vi "Load Settings from XML.vi"() -> (0 "error out":errorcluster, 3 "Settings Out":T1 {"Units" items=["degC", "degF", "kelvin", "raw"]})   [LabVIEW 2020, in "Settings Editor.lvlib"]
doc: "Attempts to load previous user specified settings from an XML file.\n\nThis VI will not generate an error. If a suitable XML file can't be loaded and parsed then it will simply return the default settings.\n_____\nBased on Delacor QMH Project Template 5.0.0.82."
uses:
  Settings Editor.lvlib
  Settings--cluster.ctl
  <vilib>/Utility/xml.llb/Read From XML File(string).vi
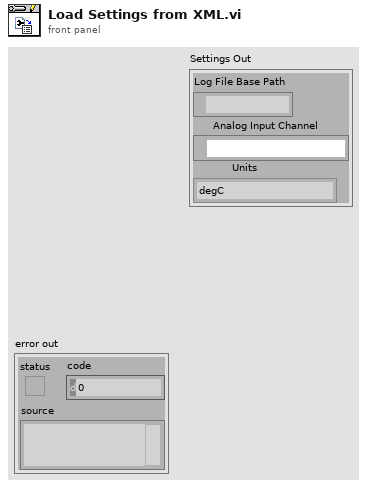
[diagram p1: front panel]
types:
  T1 = typedef "Settings Editor.lvlib/Settings--cluster.ctl" = cluster{"Log File Base Path":path, "Analog Input Channel":refnum<k21>, "Units":i32}
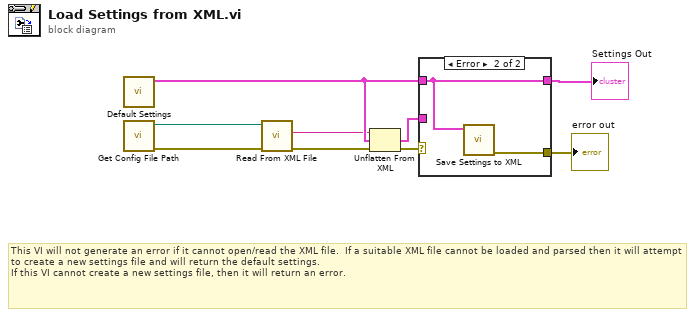
[diagram p0: block diagram]
diagram:
  # "This VI will not generate an error if it cannot open/read the XML file.  If a suitable XML file cannot be loaded and parsed then it will attempt to create a new settings file and will return the default settings.\nIf this VI cannot create a new settings file, then it will return an error."
  n1 = call "Default Settings.vi"() -> ("Default Settings"=w8:T1)  [unwired: 11 in]
  n2 = call "Get Config File Path.vi"() -> ("error out"=w4:errorcluster, "XML File Path"=w5:path)  [unwired: 10 in]
  n3 = call-poly <vilib>:"Read From XML File.vi"("error in (no error)"=w4, "XML File Path"=w5) -> ("error out"=w6:errorcluster, "XML Elements"=w7:string)  [unwired: 7 in, 1 out]
  n4 = Unflatten From XML(xml string=w7, type=w8, error in (no error)=w6) -> (value=w2:T1, error out=w3:errorcluster)
  n5 = case shown="Error" w3 {
    tunnel: [w10 w12] -> w1
    tunnel: w8 -> [_ w12]
    tunnel: w2 -> [w10 _]
    tunnel: [_ w11] -> w9
    frame No Error {
    }
    frame Error {
      n6 = call "Save Settings to XML.vi"("Settings"=w12) -> ("error out"=w11:errorcluster)  [unwired: 10 in]
    }
  }
  "error out" <- w9
  "Settings Out" <- w1
